vi "Insert Value (Single String).vi"(7 "key":string, 8 "error in (no error)":errorcluster, 10 "value":string, 11 "JSON Value in":refnum<class "JSON Value.lvclass">) -> (0 "error out":errorcluster, 1 "replaced":bool, 3 "JSON Value out":refnum<class "JSON Value.lvclass">)   [LabVIEW 2016, in "JSON Value.lvclass"]
uses:
  JSON Helper/JSON Value.lvclass
  JSON String/New JSON String.vi
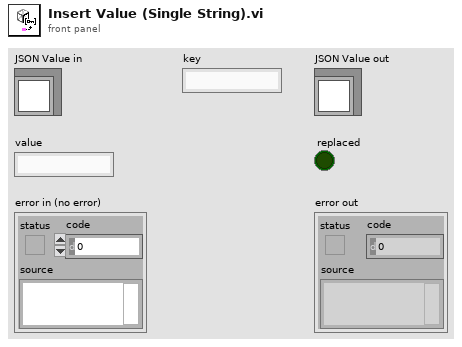
[diagram p1: front panel]
types:
  T1 = typedef "JSON Value.lvclass/JSON Types.ctl" = enum16{"String", "Numeric", "Boolean", "NULL", "Object", "Array"}
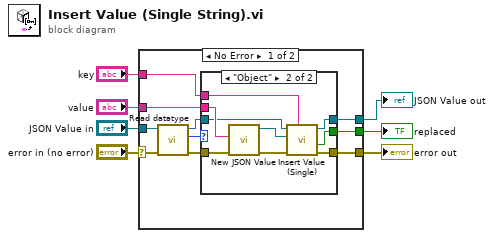
[diagram p0: block diagram]
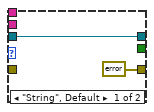
[diagram p2: hidden frame]
diagram:
  n1 = case shown="No Error" "error in (no error)" {
    selector: "error in (no error)" -> [w12 w30]
    tunnel: [w14 w30] -> w6
    tunnel: [w17 w29] -> w4
    tunnel: "JSON Value in" -> [w10 w29]
    tunnel: "key" -> [w16 _]
    tunnel: "value" -> [w15 _]
    tunnel: [w13 _] -> w1
    frame No Error {
      n2 = call "Read datatype.vi"("error in (no error)"=w12, "JSON Value in"=w10) -> ("error out"=w11:errorcluster, "datatype"=w8:T1, "JSON Value out"=w9:refnum<class "JSON Value.lvclass">)  [unwired: 7 in]
      n3 = case shown="\"Object\"" w8 {
        tunnel: [w19 w25] -> w17
        tunnel: w16 -> [_ w21]
        tunnel: w15 -> [_ w28]
        tunnel: [errorcluster {"status"=TRUE, "code"=-1000, "source"="Attempted insert on non-object"} ("error out") w22] -> w14
        tunnel: [_ w24] -> w13
        tunnel: w9 -> [w19 w26]
        tunnel: w11 -> [_ w27]
        frame "String", Default {
        }
        frame "Object" {
          n4 = call-poly "New JSON Value.vi"("error in (no error)"=w27, "value"=w28) -> ("error out"=w23:errorcluster, "JSON Value out"=w20:refnum<class "JSON Value.lvclass">)  [unwired: 8 in]
          n5 = call "Insert Value (Single).vi"("key"=w21, "error in (no error)"=w23, 10:"JSON Value in"=w20, 11:"JSON Value in"=w26) -> ("error out"=w22:errorcluster, "replaced"=w24:bool, "JSON Value out"=w25:refnum<class "JSON Value.lvclass">)  [unwired: 5 in]
        }
      }
    }
    frame Error {
    }
  }
  "error out" <- w6
  "JSON Value out" <- w4
  "replaced" <- w1
